vi "Get cmd line args.vi"(8 "error in (no error)":errorcluster) -> (0 "error out":errorcluster, 1 "Arg Cnt":i32, 2 "Cmd Line Args (1-N)":string[](array[string]), 3 "Got cmd line args?":bool, 4 "arg4":string, 5 "arg1":string, 6 "arg3":string, 7 "arg2":string)   [LabVIEW 2013]
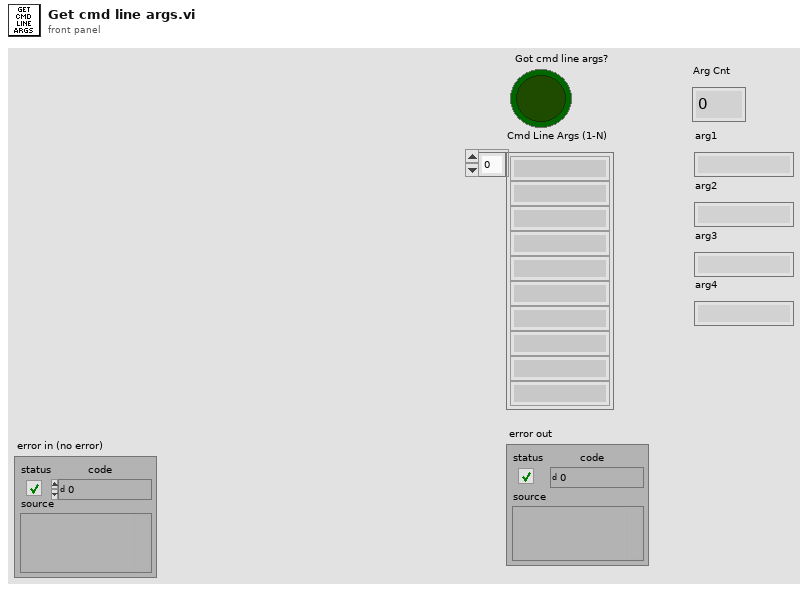
[diagram p1: front panel]
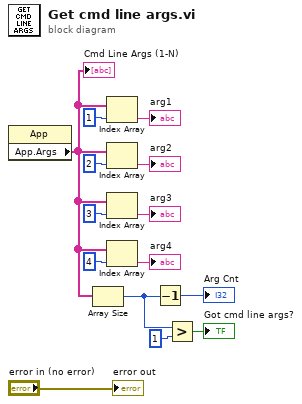
[diagram p0: block diagram]
diagram:
  n1 = property class="App"() -> ("App.Args"=w5:string[])  [unwired: 2 in, 2 out]
  "Cmd Line Args (1-N)" <- w5
  n2 = Array Size(array=w5) -> (size(s)=w11:i32)
  n3 = Index Array(array=w5, index=1) -> (element=→"arg1":string)
  n4 = Index Array(array=w5, index=2) -> (element=→"arg2":string)
  n5 = Index Array(array=w5, index=3) -> (element=→"arg3":string)
  n6 = Index Array(array=w5, index=4) -> (element=→"arg4":string)
  n7 = Decrement(x=w11) -> (x-1=→"Arg Cnt":i32)
  n8 = Greater?(x=w11, y=1) -> (0:→"Got cmd line args?":bool)
  "error out" <- "error in (no error)"
